vi "TDS DC Load Set Mode.vi"(8 "error in (no error)":errorcluster, 9 "Mode":string(combo), 10 "Signal InstConfig":string, 11 "Address":string) -> (0 "error out":errorcluster)   [LabVIEW 2025, in "Interface Functions.lvlib"]
uses:
  Interface Functions.lvlib
panel:
  # "DC Load Set Mode"
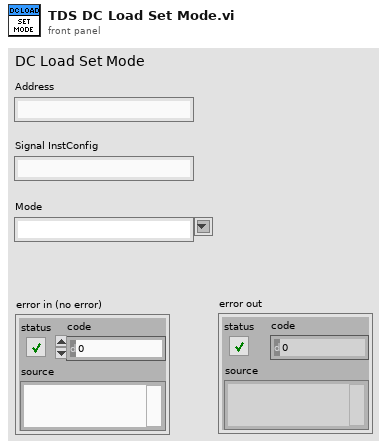
[diagram p1: front panel]
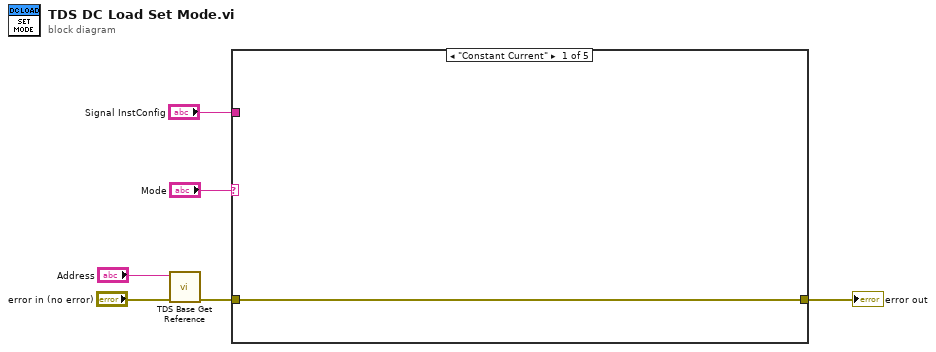
[diagram p0: block diagram]
diagram:
  n1 = call "TDS Base Get Reference.vi"("error in (no error)"="error in (no error)", "Address"="Address") -> ("error out"=w4:errorcluster)  [unwired: 8 in, 1 out]
  n2 = case shown="\"Constant Current\"" "Mode" {
    tunnel: w4 -> [w7 w8 w9 w10 w11]
    tunnel: [w7 w8 w9 w10 w11] -> w3
    tunnel: "Signal InstConfig" -> [_ _ _ _ _]
    frame "Constant Current" {
    }
    frame "Constant Voltage" {
    }
    frame "Constant Resistance" {
    }
    frame "Constant Power" {
    }
    frame "Off", Default {
    }
  }
  "error out" <- w3
